vi "HGF_SVMonitor_deregister.vi"(0 "HGF_SVMonitor in":refnum<class "HGF_SVMonitor.lvclass">, 1 "shared variable refnum":refnum<k21>, 2 "HGF_NetworkVisitor":refnum<class "HGF_NetworkVisitor.lvclass">, 3 "HGF_TriggeredEvent":refnum<class "HGF_TriggeredEvent.lvclass">, 4 "Rem SV/Visitor from List":bool, 5 "error in (no error)":errorcluster) -> (14 "HGF_SVMonitor out":refnum<class "HGF_SVMonitor.lvclass">, 19 "error out":errorcluster)   [LabVIEW 2012, in "HGF_SV.lvlib" / "HGF_SVMonitor.lvclass"]
uses:
  HGF_SVMonitor.lvclass
  HGF_BaseClasses/HGF_NetworkVisitor/HGF_NetworkVisitor.lvclass
  HGF_BaseClasses/HGF_TriggeredEvent/HGF_TriggeredEvent.lvclass
  HGF_SVMonitor.lvclass/HGF_SVMonitor.ctl
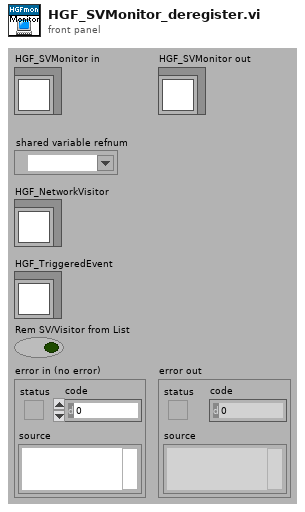
[diagram p1: front panel]
types:
  T1 = cluster{"registered Visitors":cluster{"HGF_NetworkVisitor":refnum<class "HGF_NetworkVisitor.lvclass">, "HGF_TriggeredEvent":refnum<class "HGF_TriggeredEvent.lvclass">}[], "last known data":variant, "Time Stamp":timestamp, "shared variable refnum in":refnum<k21>}[]
  T2 = cluster{"HGF_NetworkVisitor":refnum<class "HGF_NetworkVisitor.lvclass">, "HGF_TriggeredEvent":refnum<class "HGF_TriggeredEvent.lvclass">}
  T3 = cluster{"registered Visitors":cluster{"HGF_NetworkVisitor":refnum<class "HGF_NetworkVisitor.lvclass">, "HGF_TriggeredEvent":refnum<class "HGF_TriggeredEvent.lvclass">}[], "last known data":variant, "Time Stamp":timestamp, "shared variable refnum in":refnum<k21>}
  T4 = cluster{"HGF_NetworkVisitor":refnum<class "HGF_NetworkVisitor.lvclass">, "HGF_TriggeredEvent":refnum<class "HGF_TriggeredEvent.lvclass">}[]
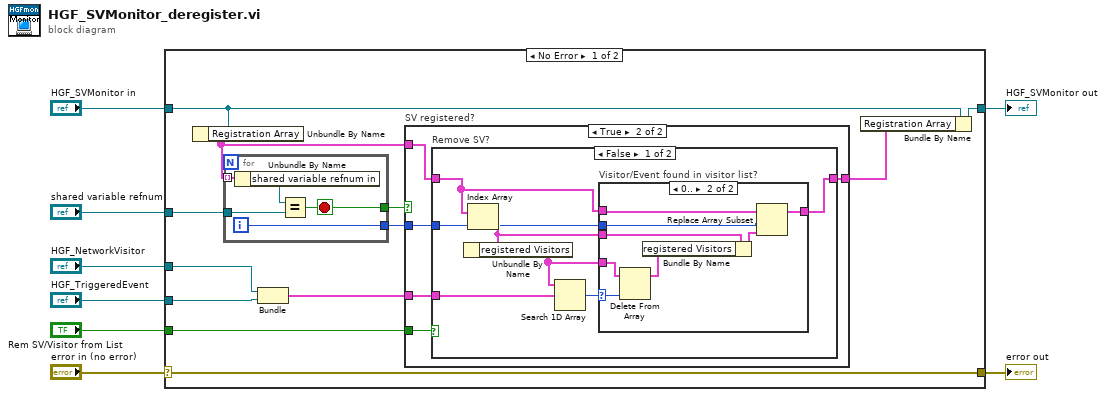
[diagram p0: block diagram]
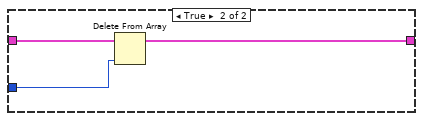
[diagram p4: hidden frame]
diagram:
  n1 = case shown="No Error" "error in (no error)" {
    selector: "error in (no error)" -> [w9 w52]
    tunnel: [w9 w52] -> w7
    tunnel: [w14 w51] -> w5
    tunnel: "HGF_SVMonitor in" -> [w20 w51]
    tunnel: "shared variable refnum" -> [w19 _]
    tunnel: "HGF_NetworkVisitor" -> [w12 _]
    tunnel: "HGF_TriggeredEvent" -> [w11 _]
    tunnel: "Rem SV/Visitor from List" -> [w17 _]
    frame No Error {
      n2 = Unbundle By Name(w20) -> ("Registration Array"=w16:T1)
      n3 = for {
        tunnel: w16 -> [w50] mode=indexing
        tunnel: w19 -> [w49]
        tunnel: [w47] -> w18
        tunnel: [w46] -> w15
        i -> [w46]
        stop <- w47 stop-if-true
        n4 = Unbundle By Name(w50) -> ("shared variable refnum in"=w48:refnum<k21>)
        n5 = Equal?(x=w48, y=w49) -> (x = y?=w47:bool)
      }
      n6 = Bundle("HGF_NetworkVisitor"=w12, "HGF_TriggeredEvent"=w11) -> (w10:T2)  [unwired: 1 in]
      n7 = case "SV registered?" shown="True" w18 {
        tunnel: w17 -> [_ w26]
        tunnel: w16 -> [w21 w25]
        tunnel: w15 -> [_ w24]
        tunnel: [w21 w23] -> w13
        tunnel: w10 -> [_ w22]
        frame False {
        }
        frame True {
          n8 = case "Remove SV?" shown="False" w26 {
            tunnel: w25 -> [w29 w45]
            tunnel: w24 -> [w28 w44]
            tunnel: [w27 w43] -> w23
            tunnel: w22 -> [w33 _]
            frame False {
              n9 = Index Array(array=w29, index=w28) -> (element=w30:T3)
              n10 = Unbundle By Name(w30) -> ("registered Visitors"=w31:T4)
              n11 = Search 1D Array(1D array=w31, element=w33) -> (index of element=w32:i32)  [unwired: 1 in]
              n12 = case "Visitor/Event found in visitor list?" shown="0.." w32 {
                selector: w32 -> [_ w42]
                tunnel: w31 -> [_ w41]
                tunnel: w30 -> [_ w40]
                tunnel: w29 -> [w34 w38]
                tunnel: w28 -> [_ w37]
                tunnel: [w34 w35] -> w27
                frame Default {
                }
                frame 0.. {
                  n13 = Delete From Array(array=w41, index=w42) -> (array with subset deleted=w39:T4)  [unwired: 1 in, 1 out]
                  n14 = Bundle By Name(cluster=w40, "registered Visitors"=w39) -> (w36:T3)
                  n15 = Replace Array Subset(array=w38, new element=w36, index=w37) -> (w35:T1)
                }
              }
            }
            frame True {
              n16 = Delete From Array(array=w45, index=w44) -> (array with subset deleted=w43:T1)  [unwired: 1 in, 1 out]
            }
          }
        }
      }
      n17 = Bundle By Name(cluster=w20, "Registration Array"=w13) -> (w14:refnum<class "HGF_SVMonitor.lvclass">)
    }
    frame Error {
    }
  }
  "error out" <- w7
  "HGF_SVMonitor out" <- w5
